vi "Read Timestamp.vi"(7 "field name":string="timeStamp", 8 "error in":errorcluster, 9 "user tag in":i32, 10 "timestamp in":timestamp, 11 "PV Data in":refnum<class "PV Data.lvclass">) -> (0 "error out":errorcluster, 1 "user tag":i32, 2 "timestamp":timestamp, 3 "PV Data out":refnum<class "PV Data.lvclass">)   [LabVIEW 2020, in "PV Access.lvlib" / "PV Data.lvlib" / "PV Data.lvclass"]
uses:
  PV Data.lvclass
  PV Access.lvlib
  PV Data.lvlib
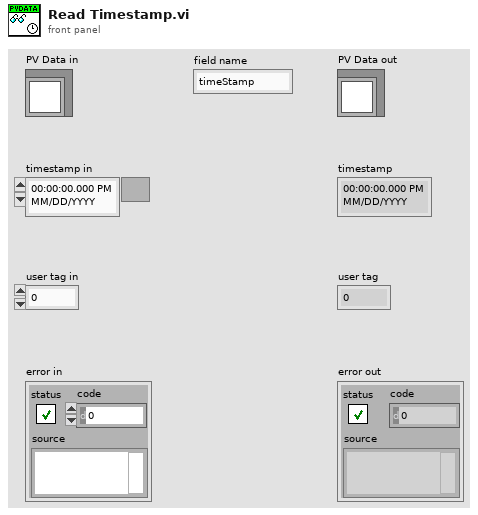
[diagram p1: front panel]
types:
  T1 = typedef "PV Access.lvlib/PV Data.lvlib/EPICS Timestamp.ctl" = cluster{"Seconds Past Epoch":i64, "Nanoseconds":i32, "User Tag":i32}
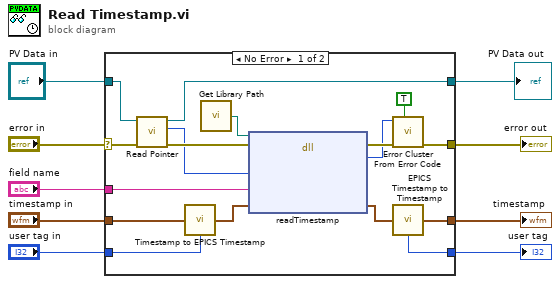
[diagram p0: block diagram]
diagram:
  n1 = case shown="No Error" "error in" {
    selector: "error in" -> [w21 w28]
    tunnel: [w22 w28] -> w9
    tunnel: "PV Data in" -> [w19 w27]
    tunnel: [w17 w27] -> w6
    tunnel: "field name" -> [w16 _]
    tunnel: [w14 _] -> w4
    tunnel: [w13 _] -> w3
    tunnel: "timestamp in" -> [w11 _]
    tunnel: "user tag in" -> [w10 _]
    frame No Error {
      n2 = call-dynamic "Read Pointer.vi"("error in (no error)"=w21, "Pointer Base in"=w19) -> ("error out"=w20:errorcluster, "Pointer"=w18:i64, "Pointer Base out"=w17:refnum<class "PV Data.lvclass">)  [unwired: 7 in]
      n3 = call "Timestamp to EPICS Timestamp.vi"("timestamp"=w11, "user tag"=w10) -> ("epics timestamp"=w12:T1)
      n4 = call "Get Library Path.vi"() -> ("Path"=w26:path)  [unwired: 1 in]
      n5 = dll-call lib="?" fn="readTimestamp"(path in=w26, error in=w20, "value"=w18, "field_name"=w16, "EPICS timestamp"=w12) -> (error out=w24:errorcluster, "err_code"=w23:i32, "EPICS timestamp"=w15:T1)  [unwired: 3 in, 1 out]
      n6 = call <vilib>:"Error Cluster From Error Code.vi"("show call chain? (False)"=TRUE, "error in (no error)"=w24, "error code (0)"=w23) -> ("error out"=w22:errorcluster)  [unwired: 6 in]
      n7 = call "EPICS Timestamp to Timestamp.vi"("EPICS timestamp"=w15) -> ("user tag"=w14:i32, "timestamp"=w13:timestamp)
    }
    frame Error {
    }
  }
  "error out" <- w9
  "PV Data out" <- w6
  "timestamp" <- w3
  "user tag" <- w4
